vi "New Project.vi"(9 "DBSet":T1={"Server"="172.20.23.107", "DB"="HTPSDB", "PSW"="data'songyy", "User"="sa"}, 10 "UserID":string="L043460", 11 "厂区":string="清溪") -> ()   [LabVIEW 2011] (continued)
      n38 = call "Delete empty element from array.vi"("Array In"=w75) -> ("Array out"=w39:string[])  [unwired: 26 in]
      "Single init" <- w39
      n39 = call "Delete empty element from array.vi"("Array In"=w74) -> ("Array out"=w38:string[])  [unwired: 26 in]
      "TDR init" <- w38
      n40 = call "Delete empty element from array.vi"("Array In"=w73) -> ("Array out"=w37:string[])  [unwired: 26 in]
      "S-p init" <- w37
      n41 = call "Delete empty element from array.vi"("Array In"=w72) -> ("Array out"=w36:string[])  [unwired: 26 in]
      "NEXT init" <- w36
      n42 = call "Delete empty element from array.vi"("Array In"=w64) -> ("Array out"=w35:string[])  [unwired: 26 in]
      "FEXT init" <- w35
      n43 = Array Size(array=w69) -> (size(s)=w90:i32)
      n44 = Array Size(array=w39) -> (size(s)=w87:i32)
      n45 = Array Size(array=w38) -> (size(s)=w63:i32)
      n46 = Array Size(array=w37) -> (size(s)=w70:i32)
      n47 = Array Size(array=w36) -> (size(s)=w88:i32)
      n48 = Array Size(array=w35) -> (size(s)=w71:i32)
      n49 = property on="Postion for Raw data" class="Tbl (严格)"("Value"=string[][] [] ("Postion for Raw data")) -> ()  [unwired: 2 in, 2 out]
      n50 = Initialize Array(w62, w90) -> (w54:i32[])
      "Diff init" <- w54
      n51 = Initialize Array(w62, w87) -> (w53:i32[])
      "Single init" <- w53
      n52 = Initialize Array(w62, w63) -> (w52:i32[])
      "TDR init" <- w52
      n53 = Initialize Array(w62, w70) -> (w89:i32[])
      "S-p init" <- w89
      n54 = Initialize Array(w62, w88) -> (w51:i32[])
      "NEXT init" <- w51
      n55 = Initialize Array(w62, w71) -> (w50:i32[])
      "FEXT init" <- w50
      n56 = property on="Diff Test Items" class="LstBox (严格)"("Item Names"=w69, "Item Symbols"=w54) -> ()  [unwired: 2 in, 2 out]
      n57 = property on="Single Test Items" class="LstBox (严格)"("Item Names"=w39, "Item Symbols"=w53) -> ()  [unwired: 2 in, 2 out]
      n58 = property on="TDR Test Items" class="LstBox (严格)"("Item Names"=w38, "Item Symbols"=w52) -> ()  [unwired: 2 in, 2 out]
      n59 = property on="S-para Pair Name" class="LstBox (严格)"("Item Names"=w37, "Item Symbols"=w89) -> ()  [unwired: 2 in, 2 out]
      n60 = property on="NEXT Pair Name" class="LstBox (严格)"("Item Names"=w36, "Item Symbols"=w51) -> ()  [unwired: 2 in, 2 out]
      n61 = property on="FEXT Pair Name" class="LstBox (严格)"("Item Names"=w35, "Item Symbols"=w50) -> ()  [unwired: 2 in, 2 out]
      n62 = property on="访问DB(s)" class="DigNum (严格)"("Visible"=TRUE ("可见")) -> ()  [unwired: 2 in, 2 out]
      n63 = local write "fre-save"(string[] [] ("fre-save")) -> ()
      n64 = Get Date/Time In Seconds() -> (seconds since 1Jan1904=→"midVar_timeStart":timestamp)
      n65 = local write "EEPROM Write/Read ?"(w60) -> ()
      n66 = local write "Label Print?"(w60) -> ()
      n67 = local write "Report Templete Path:"(path "" ("Report Templete Path:")) -> ()
      n68 = property on="Postion for \"PN&Tester&Date\" etc Fields" class="Tbl (严格)"("Value"=string[][] [["Applicant", "0", "2", "1"], ["Part Name", "0", "3", "1"], ["Part Number", "0", "4", "1"], ["Report No", "0", "2", "12"], ["Sample No", "0", "4", "12"], ["Prepared By", "0", "63", "0"], ["Approved By", "0", "63", "6"], ["Date", "0", "63", "2"], ["Thru Result", "0", "13", "5"], ["NEXT Result", "0", "45", "4"], ["FEXT Result", "0", "45", "5"]] ("Postion for \"PN&Tester&Date\" etc Fields")) -> ()  [unwired: 2 in, 2 out]
      n69 = property on="Postion for Raw data" class="Tbl (严格)"("Number of Columns"=w59, "EditPos"=w58) -> ()  [unwired: 2 in, 2 out]
      n70 = property on="Postion for \"PN&Tester&Date\" etc Fields" class="Tbl (严格)"("Number of Columns"=w59, "EditPos"=w58) -> ()  [unwired: 2 in, 2 out]
      n71 = local write "Spec Points"(1601.0 ("Spec Points")) -> ()
      n72 = local write "Quick"(FALSE ("Quick")) -> ()
      n73 = local write "Spec Associate"(string[][] [] ("Spec Associate")) -> ()
      n74 = property on="Diff Test Items" class="LstBox (严格)"("Value"=w57) -> ()  [unwired: 2 in, 2 out]
      n75 = property on="S-para Pair Name" class="LstBox (严格)"("Value"=w57) -> ()  [unwired: 2 in, 2 out]
      n76 = property on="NEXT Pair Name" class="LstBox (严格)"("Value"=w57) -> ()  [unwired: 2 in, 2 out]
      n77 = property on="FEXT Pair Name" class="LstBox (严格)"("Value"=w57) -> ()  [unwired: 2 in, 2 out]
      n78 = property on="Single Test Items" class="LstBox (严格)"("Value"=w57) -> ()  [unwired: 2 in, 2 out]
      n79 = property on="FEXT Pair Name" class="LstBox (严格)"("Value"=w57) -> ()  [unwired: 2 in, 2 out]
      n80 = property on="Cable AWG:" class="Ring (严格)"("Value"=w57) -> ()  [unwired: 2 in, 2 out]
      n81 = property on="Customer" class="Ring (严格)"("Value"=w57) -> ()  [unwired: 2 in, 2 out]
      n82 = property on="TDR Test Items" class="LstBox (严格)"("Value"=w57) -> ()  [unwired: 2 in, 2 out]
      n83 = call <vilib>:"Application Directory.vi"() -> ("Application Directory"=w33:path)
      n84 = property on="Default" class="RadioBtnsControl (严格)"("Value"=w57) -> ()  [unwired: 2 in, 2 out]
      n85 = Build Path(base path=w33, name or relative path="template" ("名称或相对路径")) -> (appended path=w34:path)
      n86 = call "Get_initialize_Config.vi"() -> ("Local Database"=w25:bool)  [unwired: 11 in]
      n87 = local write "Report Templete Path:"(w34) -> ()
      n88 = local write "Local"(w25) -> ()
      n89 = property on="Excute" class="Bool"("DisabledEnum"=w30) -> ()  [unwired: 2 in, 2 out]
      n90 = property on="Query" class="Bool (严格)"("DisabledEnum"=w30) -> ()  [unwired: 2 in, 2 out]
      n91 = property on="Save" class="Bool (严格)"("DisabledEnum"=T5."Disabled and Grayed Out" ("禁用")) -> ()  [unwired: 2 in, 2 out]
      n92 = local write "Save"(FALSE ("Query")) -> ()
      n93 = local write "Delete"(FALSE ("Query")) -> ()
      n94 = local write "Query"(FALSE ("Query")) -> ()
      n95 = local write "Update"(FALSE ("Query")) -> ()
      n96 = property on="SNType" class="Str"("Visible"=w25) -> ()  [unwired: 2 in, 2 out]
      n97 = property on="CmdType" class="Ring (严格)"("Visible"=w25) -> ()  [unwired: 2 in, 2 out]
      n98 = property on="Update" class="Bool (严格)"("DisabledEnum"=T5."Disabled and Grayed Out" ("禁用")) -> ()  [unwired: 2 in, 2 out]
      n99 = property on="Delete" class="Bool (严格)"("DisabledEnum"=T5."Disabled and Grayed Out" ("禁用")) -> ()  [unwired: 2 in, 2 out]
      n100 = property on="Luxshare_P/N:" class="Str"("DisabledEnum"=T5."Disabled and Grayed Out" ("禁用")) -> ()  [unwired: 2 in, 2 out]
      "midVar_bool_timStop" <- FALSE ("midVar_bool_timStop")
    }
    frame #2 {
      n101 = while {
        stop <- w103 stop-if-true
        n102 = local read "midVar_timeStart"() -> (w102:timestamp)
        n103 = local read "midVar_bool_timStop"() -> (w103:bool)
        n104 = Get Date/Time In Seconds() -> (seconds since 1Jan1904=w104:timestamp)
        n105 = Subtract(x=w104, y=w102) -> (x-y=→"访问DB(s)":dbl)
      }
      n106 = call <vilib>:"System Exec.vi"("run minimized? (F)"=TRUE, "wait until completion? (T)"=TRUE, "command line"="ping DG-MESDB.luxshare.com.cn") -> ("standard output"=w95:string)  [unwired: 5 in, 3 out]
      n107 = Search and Replace String(replace all?=TRUE ("替换全部？(F)"), case sensitive?=TRUE ("忽略大小写？(F)"), input string=w95, search string="TTL" ("搜索字符串")) -> (number of replacements=w97:i32)  [unwired: 4 in, 3 out]
      n108 = Greater Than 0?(x=w97) -> (x > 0?=w92:bool)
      n109 = case shown="真" w92 {
        tunnel: "DBSet" -> [_ w112]
        frame False {
          w108 = T5."Enabled" ("禁用")
          # "连不上数据库，local禁用，默认勾选"
          n110 = property on="Query" class="Bool (严格)"("DisabledEnum"=w108) -> ()  [unwired: 2 in, 2 out]
          n111 = property on="Save" class="Bool (严格)"("DisabledEnum"=w108) -> ()  [unwired: 2 in, 2 out]
          n112 = local write "midVar_bool_timStop"(TRUE ("midVar_bool_timStop")) -> ()
          n113 = One Button Dialog(message="fail to connect DB!\nyou can use local DB only!") -> ()  [unwired: 1 in, 1 out]
          n114 = property on="Excute" class="Bool"("DisabledEnum"=w108) -> ()  [unwired: 2 in, 2 out]
          n115 = local write "Local"(TRUE ("Local")) -> ()
          n116 = property on="Local" class="Bool (严格)"("DisabledEnum"=T5."Disabled and Grayed Out" ("禁用")) -> ()  [unwired: 2 in, 2 out]
          n117 = property on="FixtureNo" class="CmbBox"("Strings And Values[]"=T6 [{"String"="No Data", "Value"="No Data"}] ("字符串与值[]")) -> ()  [unwired: 2 in, 2 out]
          n118 = property on="FixtureNo" class="CmbBox"("DisabledEnum"=T5."Disabled and Grayed Out" ("禁用")) -> ()  [unwired: 2 in, 2 out]
        }
        frame True {
          n119 = stacked-sequence {
            tunnel: w112 -> [_ w115 _]
            frame #0 {
              w114 = T5."Enabled" ("禁用")
              w113 = T5."Enabled" ("禁用")
              n120 = property on="Local" class="Bool (严格)"("DisabledEnum"=w113) -> ()  [unwired: 2 in, 2 out]
              n121 = property on="Query" class="Bool (严格)"("DisabledEnum"=w113) -> ()  [unwired: 2 in, 2 out]
              n122 = property on="Save" class="Bool (严格)"("DisabledEnum"=w114) -> ()  [unwired: 2 in, 2 out]
              n123 = property on="Excute" class="Bool"("DisabledEnum"=w114) -> ()  [unwired: 2 in, 2 out]
            }
            frame #1 {
              n124 = disable-structure shown="禁用" {
                disable-tunnel: w115 -> [w116 _]
                frame Disabled {
                  n125 = call "sql-readinfo_vproject.vi"("DBSet"=w116, "操作模式"=T7."查询数据", "查询项目"="FixtureNo", "限定条件"="") -> ("ConvertToArray"=w118:string[][], "ResultString"=w117:string)  [unwired: 13 in, 9 out]
                  n126 = call <vilib>:"Trim Whitespace.vi"("string"=w117) -> ("trimmed string"=w123:string)  [unwired: 1 in]
                  n127 = Empty String/Path?(string/path=w123) -> (empty?=w122:bool)
                  n128 = case shown="假" w122 {
                    tunnel: w118 -> [w128 _]
                    frame False {
                      n129 = Index Array(array=w128, index (col)=0 ("索引 (行)")) -> (element=w127:string[])  [unwired: 1 in]
                      n130 = for {
                        tunnel: w127 -> [w130] mode=indexing
                        tunnel: [w129] -> w126 mode=indexing
                        n131 = Bundle("字符串"=w130, "字符串"=w130) -> (w129:cluster{"字符串":string, "字符串":string})  [unwired: 1 in]
                      }
                      n132 = property on="FixtureNo" class="CmbBox"("Strings And Values[]"=w126) -> ()  [unwired: 2 in, 2 out]
                      n133 = property on="FixtureNo" class="CmbBox"("DisabledEnum"=T5."Enabled" ("禁用")) -> ()  [unwired: 2 in, 2 out]
                    }
                    frame True {
                      n134 = property on="FixtureNo" class="CmbBox"("Strings And Values[]"=T6 [{"String"="No Data", "Value"="No Data"}] ("字符串与值[]")) -> ()  [unwired: 2 in, 2 out]
                      n135 = property on="FixtureNo" class="CmbBox"("DisabledEnum"=T5."Disabled and Grayed Out" ("禁用")) -> ()  [unwired: 2 in, 2 out]
                    }
                  }
                }
                frame Enabled {
                }
              }
            }
            frame #2 {
              n136 = local write "midVar_bool_timStop"(TRUE ("midVar_bool_timStop")) -> ()
            }
          }
        }
      }
    }
    frame #3 {
      n137 = control-ref of="Label Num"() -> (w141:refnum<vi>)
      n138 = control-ref of="FixtureNo"() -> (w163:refnum<vi>)
      n139 = control-ref of="Label Num"() -> (w162:refnum<vi>)
      n140 = control-ref of="Label Content"() -> (w161:refnum<vi>)
      n141 = control-ref of="SNType"() -> (w160:refnum<vi>)
      n142 = control-ref of="Customer_P/N:"() -> (w170:refnum<vi>)
      n143 = control-ref of="Length(mm):"() -> (w169:refnum<vi>)
      n144 = control-ref of="Sample Description:"() -> (w168:refnum<vi>)
      n145 = control-ref of="Remark:"() -> (w167:refnum<vi>)
      n146 = control-ref of="Switch Matrix"() -> (w166:refnum<vi>)
      n147 = control-ref of="VNA Cal File Path:"() -> (w164:refnum<vi>)
      n148 = control-ref of="EEPROM Write/Read ?"() -> (w159:refnum<vi>)
      n149 = control-ref of="Label Print?"() -> (w158:refnum<vi>)
      n150 = Build Array(w159, w158) -> (→"bool":refnum<vi>[])
      n151 = call <vilib>:"Application Directory.vi"() -> ("Application Directory"=w137:path)
      n152 = Build Array(w164, w170, w169, w168, w167, w166, w163, w162, w161, w141, w160) -> (→"string":refnum<vi>[])
      n153 = Build Path(base path=w137, name or relative path="Database" ("名称或相对路径")) -> (appended path=w140:path)
      n154 = Build Path(base path=w140, name or relative path="FigoConfig.xml" ("名称或相对路径")) -> (appended path=w136:path)
      n155 = control-ref of="Postion for Raw data"() -> (w156:refnum<vi>)
      n156 = control-ref of="Impedance Spec:"() -> (w142:refnum<vi>)
      n157 = control-ref of="Start TimeNs"() -> (w155:refnum<vi>)
      n158 = control-ref of="StopTimeNs"() -> (w154:refnum<vi>)
      n159 = control-ref of="Filter Risetime(ps)"() -> (w153:refnum<vi>)
      n160 = control-ref of="Compensation(ohm)"() -> (w152:refnum<vi>)
      n161 = call <vilib>:"Check if File or Folder Exists.vi"("path"=w136) -> ("file or folder exists?"=w135:bool, "dup path"=w134:path)  [unwired: 8 in, 1 out]
      n162 = Build Array(w142, w156) -> (→"chart":refnum<vi>[])
      n163 = Build Array(w155, w154, w153, w152) -> (→"number":refnum<vi>[])
      n164 = case shown="真" w135 {
        tunnel: w134 -> [_ w173]
        frame False {
        }
        frame True {
          n165 = call "xmlConfigRead.vi"("path to XML document"=w173, "XPath expression"="//AWG/item/@value") -> ("OutParaArray"=w172:string[])  [unwired: 2 out]
          n166 = property on="Cable AWG:" class="Ring (严格)"("Strings []"=w172) -> ()  [unwired: 2 in, 2 out]
        }
      }
      n167 = control-ref of="Diff Test Items"() -> (w151:refnum<vi>)
      n168 = control-ref of="Single Test Items"() -> (w150:refnum<vi>)
      n169 = control-ref of="TDR Test Items"() -> (w149:refnum<vi>)
      n170 = control-ref of="S-para Pair Name"() -> (w148:refnum<vi>)
      n171 = control-ref of="NEXT Pair Name"() -> (w147:refnum<vi>)
      n172 = control-ref of="FEXT Pair Name"() -> (w146:refnum<vi>)
      n173 = Build Array(w151, w150, w149, w148, w147, w146) -> (→"list":refnum<vi>[])
      n174 = property on="访问DB(s)" class="DigNum (严格)"("Visible"=FALSE ("可见")) -> ()  [unwired: 2 in, 2 out]
    }
    frame #4 {
      n175 = while {
        stop <- w176 stop-if-true
        n176 = event shown="[17] \"Excute\": 值改变" {
          selector: _ -> [_ _ _ _ _ _ _ _ _ _ _ _ _ _ _ _ _ _ _ _ _ _ _]
          dyn-events: _ -> [_ _ _ _ _ _ _ _ _ _ _ _ _ _ _ _ _ _ _ _ _ _ _]
          timeout: 500 -> [_ _ _ _ _ _ _ _ _ _ _ _ _ _ _ _ _ _ _ _ _ _ _]
          tunnel: [_ _ _ _ _ _ _ _ _ _ _ _ _ _ _ _ _ _ _ TRUE _ _ _] -> w176
          event Timeout {
            n177 = event-data() -> ()  [unwired: 1 in, 2 out]
          }
          event "Length(mm):", "VNA Cal File Path:", "Switch Matrix", "Luxshare_P/N:": Value Change {
            n178 = event-data() -> ()  [unwired: 1 in, 5 out]
          }
          event "Local": Value Change {
            n179 = event-data() -> ()  [unwired: 1 in, 5 out]
            n180 = local read "Local"() -> (w177:bool)
            n181 = Not(x=w177) -> (.not. x?=w178:bool)
            n182 = property on="SNType" class="Str"("Visible"=w177) -> ()  [unwired: 2 in, 2 out]
            n183 = property on="CmdType" class="Ring (严格)"("Visible"=w177) -> ()  [unwired: 2 in, 2 out]
            n184 = property on="System_Mode" class="Ring (严格)"("Visible"=w178) -> ()  [unwired: 2 in, 2 out]
          }
          event "Quick": Value Change {
            n185 = event-data() -> ("NewVal"=w181:bool)  [unwired: 1 in, 4 out]
            n186 = Equal?(x=w181, y=TRUE) -> (x = y?=w179:bool)
            n187 = case shown="真" w179 {
              frame False {
                n188 = property on="Postion for Raw data" class="Tbl (严格)"("Value"=string[][] [] ("Postion for Raw data")) -> ()  [unwired: 2 in, 2 out]
              }
              frame True {
                w184 = T4 {"Row"=0, "Column"=0} ("编辑位置")
                w185 = u32 4 ("列数")
                n189 = property on="Single Test Items" class="LstBox (严格)"() -> ("Item Names"=w202:string[], "Item Symbols"=w201:i32[])  [unwired: 2 in, 2 out]
                n190 = property on="TDR Test Items" class="LstBox (严格)"() -> ("Item Names"=w200:string[], "Item Symbols"=w199:i32[])  [unwired: 2 in, 2 out]
                n191 = property on="Diff Test Items" class="LstBox (严格)"() -> ("Item Names"=w204:string[], "Item Symbols"=w203:i32[])  [unwired: 2 in, 2 out]
                n192 = call "_wmg_SelectItems2.vi"("Item Syms"=w199, "Item name"=w200) -> ("Selected tem"=w198:string[])  [unwired: 7 in, 2 out]
                n193 = call "_wmg_SelectItems2.vi"("Item Syms"=w203, "Item name"=w204) -> ("Selected tem"=w197:string[])  [unwired: 7 in, 2 out]
                n194 = call "_wmg_SelectItems2.vi"("Item Syms"=w201, "Item name"=w202) -> ("Selected tem"=w196:string[])  [unwired: 7 in, 2 out]
                n195 = Insert Into Array(array=w198, new element #1=w197, new element #2=w196) -> (w193:string[])  [unwired: 1 in]
                n196 = Array Size(array=w193) -> (size(s)=w190:i32)
                n197 = for {
                  N: w190 -> [_]
                  tunnel: [w205] -> w194 mode=indexing
                  i -> [w206]
                  n198 = Increment(x=w206) -> (x+1=w205:i32)
                }
                n199 = Initialize Array("2", w190) -> (w188:string[])
                n200 = Initialize Array("0", w190) -> (w187:string[])
                n201 = Number To Decimal String(number=w194) -> (decimal integer string=w192:string[])  [unwired: 1 in]
                n202 = Build Array(w193, w192, w188, w187) -> (w186:string[][])
                n203 = Transpose 2D Array(2D array=w186) -> (transposed array=w195:string[][])
                n204 = property on="Postion for Raw data" class="Tbl (严格)"("Value"=w195, "EditPos"=T4 {"Row"=0, "Column"=0} ("编辑位置")) -> ()  [unwired: 2 in, 2 out]
                n205 = property on="Postion for Raw data" class="Tbl (严格)"("Number of Columns"=w185, "EditPos"=w184) -> ()  [unwired: 2 in, 2 out]
                n206 = property on="Postion for \"PN&Tester&Date\" etc Fields" class="Tbl (严格)"("Number of Columns"=w185, "EditPos"=w184) -> ()  [unwired: 2 in, 2 out]
              }
            }
          }
          event "Diff Test Items": Double Click {
            n207 = event-data() -> ("Row"=w207:i32)  [unwired: 1 in, 7 out]
            n208 = stacked-sequence {
              tunnel: w207 -> [w211 _ _]
              frame #0 {
                n209 = property on="Diff Test Items" class="LstBox (严格)"() -> ("Item Symbols"=w212:i32[])  [unwired: 2 in, 2 out]
                n210 = Index Array(array=w212, index=w211) -> (element=w209:i32)
                n211 = case shown="38" w209 {
                  tunnel: [37 38 17] -> w208
                  frame 17 {
                  }
                  frame 37, Default {
                  }
                  frame 38 {
                  }
                }
                n212 = Replace Array Subset(array=w212, new element=w208, index=w211) -> (w210:i32[])
                n213 = property on="Diff Test Items" class="LstBox (严格)"("Item Symbols"=w210) -> ()  [unwired: 2 in, 2 out]
              }
              frame #1 {
                n214 = property on="Postion for Raw data" class="Tbl (严格)"("Value"=string[][] [] ("Postion for Raw data"), "EditPos"=T4 {"Row"=0, "Column"=0} ("编辑位置")) -> ()  [unwired: 2 in, 2 out]
              }
              frame #2 {
                w219 = T4 {"Row"=0, "Column"=0} ("编辑位置")
                w220 = u32 4 ("列数")
                n215 = property on="Single Test Items" class="LstBox (严格)"() -> ("Item Names"=w237:string[], "Item Symbols"=w236:i32[])  [unwired: 2 in, 2 out]
                n216 = property on="TDR Test Items" class="LstBox (严格)"() -> ("Item Names"=w235:string[], "Item Symbols"=w234:i32[])  [unwired: 2 in, 2 out]
                n217 = property on="Diff Test Items" class="LstBox (严格)"() -> ("Item Names"=w239:string[], "Item Symbols"=w238:i32[])  [unwired: 2 in, 2 out]
                n218 = property on="Postion for Raw data" class="Tbl (严格)"("Number of Columns"=w220, "EditPos"=w219) -> ()  [unwired: 2 in, 2 out]
                n219 = property on="Postion for \"PN&Tester&Date\" etc Fields" class="Tbl (严格)"("Number of Columns"=w220, "EditPos"=w219) -> ()  [unwired: 2 in, 2 out]
                n220 = call "_wmg_SelectItems2.vi"("Item Syms"=w234, "Item name"=w235) -> ("Selected tem"=w233:string[])  [unwired: 7 in, 2 out]
                n221 = call "_wmg_SelectItems2.vi"("Item Syms"=w238, "Item name"=w239) -> ("Selected tem"=w232:string[])  [unwired: 7 in, 2 out]
                n222 = call "_wmg_SelectItems2.vi"("Item Syms"=w236, "Item name"=w237) -> ("Selected tem"=w231:string[])  [unwired: 7 in, 2 out]
                n223 = Insert Into Array(array=w233, new element #1=w232, new element #2=w231) -> (w228:string[])  [unwired: 1 in]
                n224 = Array Size(array=w228) -> (size(s)=w225:i32)
                n225 = for {
                  N: w225 -> [_]
                  tunnel: [w240] -> w229 mode=indexing
                  i -> [w241]
                  n226 = Increment(x=w241) -> (x+1=w240:i32)
                }
                n227 = Initialize Array("2", w225) -> (w223:string[])
                n228 = Initialize Array("0", w225) -> (w222:string[])
                n229 = Number To Decimal String(number=w229) -> (decimal integer string=w227:string[])  [unwired: 1 in]
                n230 = Build Array(w228, w227, w223, w222) -> (w221:string[][])
                n231 = Transpose 2D Array(2D array=w221) -> (transposed array=w230:string[][])
                n232 = property on="Postion for Raw data" class="Tbl (严格)"("Value"=w230, "EditPos"=T4 {"Row"=0, "Column"=0} ("编辑位置")) -> ()  [unwired: 2 in, 2 out]
              }
            }
          }
          event "TDR Test Items": Double Click {
            n233 = event-data() -> ("Row"=w242:i32)  [unwired: 1 in, 7 out]
            n234 = stacked-sequence {
              tunnel: w242 -> [w250 _ _]
              frame #0 {
                w247 = 38 ("y")
                n235 = property on="TDR Test Items" class="LstBox (严格)"() -> ("Item Symbols"=w244:i32[])  [unwired: 2 in, 2 out]
                n236 = Index Array(array=w244, index=w250) -> (element=w249:i32)
                n237 = Equal?(x=w249, y=w247) -> (x = y?=w248:bool)
                n238 = Select(t=37, s=w248, f=w247) -> (s? t:f=w245:i32)
                n239 = Replace Array Subset(array=w244, new element=w245, index=w250) -> (w243:i32[])
                n240 = property on="TDR Test Items" class="LstBox (严格)"("Item Symbols"=w243) -> ()  [unwired: 2 in, 2 out]
              }
              frame #1 {
                n241 = property on="Postion for Raw data" class="Tbl (严格)"("Value"=string[][] [] ("Postion for Raw data"), "EditPos"=T4 {"Row"=0, "Column"=0} ("编辑位置")) -> ()  [unwired: 2 in, 2 out]
              }
              frame #2 {
                w254 = T4 {"Row"=0, "Column"=0} ("编辑位置")
                w255 = u32 4 ("列数")
                n242 = property on="Single Test Items" class="LstBox (严格)"() -> ("Item Names"=w272:string[], "Item Symbols"=w271:i32[])  [unwired: 2 in, 2 out]
                n243 = property on="TDR Test Items" class="LstBox (严格)"() -> ("Item Names"=w270:string[], "Item Symbols"=w269:i32[])  [unwired: 2 in, 2 out]
                n244 = property on="Diff Test Items" class="LstBox (严格)"() -> ("Item Names"=w274:string[], "Item Symbols"=w273:i32[])  [unwired: 2 in, 2 out]
                n245 = property on="Postion for Raw data" class="Tbl (严格)"("Number of Columns"=w255, "EditPos"=w254) -> ()  [unwired: 2 in, 2 out]
                n246 = property on="Postion for \"PN&Tester&Date\" etc Fields" class="Tbl (严格)"("Number of Columns"=w255, "EditPos"=w254) -> ()  [unwired: 2 in, 2 out]
                n247 = call "_wmg_SelectItems2.vi"("Item Syms"=w269, "Item name"=w270) -> ("Selected tem"=w268:string[])  [unwired: 7 in, 2 out]
                n248 = call "_wmg_SelectItems2.vi"("Item Syms"=w273, "Item name"=w274) -> ("Selected tem"=w267:string[])  [unwired: 7 in, 2 out]
                n249 = call "_wmg_SelectItems2.vi"("Item Syms"=w271, "Item name"=w272) -> ("Selected tem"=w266:string[])  [unwired: 7 in, 2 out]
                n250 = Insert Into Array(array=w268, new element #1=w267, new element #2=w266) -> (w263:string[])  [unwired: 1 in]
                n251 = Array Size(array=w263) -> (size(s)=w260:i32)
                n252 = for {
                  N: w260 -> [_]
                  tunnel: [w275] -> w264 mode=indexing
                  i -> [w276]
                  n253 = Increment(x=w276) -> (x+1=w275:i32)
                }
                n254 = Initialize Array("2", w260) -> (w258:string[])
                n255 = Initialize Array("0", w260) -> (w257:string[])
                n256 = Number To Decimal String(number=w264) -> (decimal integer string=w262:string[])  [unwired: 1 in]
                n257 = Build Array(w263, w262, w258, w257) -> (w256:string[][])
                n258 = Transpose 2D Array(2D array=w256) -> (transposed array=w265:string[][])
                n259 = property on="Postion for Raw data" class="Tbl (严格)"("Value"=w265, "EditPos"=T4 {"Row"=0, "Column"=0} ("编辑位置")) -> ()  [unwired: 2 in, 2 out]
              }
            }
          }
          event "S-para Pair Name": Double Click {
            w281 = 38 ("y")
            n260 = event-data() -> ("Row"=w277:i32)  [unwired: 1 in, 7 out]
            n261 = property on="S-para Pair Name" class="LstBox (严格)"() -> ("Item Symbols"=w284:i32[])  [unwired: 2 in, 2 out]
            n262 = Index Array(array=w284, index=w277) -> (element=w283:i32)
            n263 = Equal?(x=w283, y=w281) -> (x = y?=w282:bool)
            n264 = Select(t=37, s=w282, f=w281) -> (s? t:f=w279:i32)
            n265 = Replace Array Subset(array=w284, new element=w279, index=w277) -> (w278:i32[])
            n266 = property on="S-para Pair Name" class="LstBox (严格)"("Item Symbols"=w278) -> ()  [unwired: 2 in, 2 out]
          }
          event "NEXT Pair Name": Double Click {
            w289 = 38 ("y")
            n267 = event-data() -> ("Row"=w285:i32)  [unwired: 1 in, 7 out]
            n268 = property on="NEXT Pair Name" class="LstBox (严格)"() -> ("Item Symbols"=w292:i32[])  [unwired: 2 in, 2 out]
            n269 = Index Array(array=w292, index=w285) -> (element=w291:i32)
            n270 = Equal?(x=w291, y=w289) -> (x = y?=w290:bool)
            n271 = Select(t=37, s=w290, f=w289) -> (s? t:f=w287:i32)
            n272 = Replace Array Subset(array=w292, new element=w287, index=w285) -> (w286:i32[])
            n273 = property on="NEXT Pair Name" class="LstBox (严格)"("Item Symbols"=w286) -> ()  [unwired: 2 in, 2 out]
          }
          event "FEXT Pair Name": Double Click {
            w293 = 38 ("y")
            n274 = event-data() -> ("Row"=w294:i32)  [unwired: 1 in, 7 out]
            n275 = property on="FEXT Pair Name" class="LstBox (严格)"() -> ("Item Symbols"=w300:i32[])  [unwired: 2 in, 2 out]
            n276 = Index Array(array=w300, index=w294) -> (element=w299:i32)
            n277 = Equal?(x=w299, y=w293) -> (x = y?=w298:bool)
            n278 = Select(t=37, s=w298, f=w293) -> (s? t:f=w296:i32)
            n279 = Replace Array Subset(array=w300, new element=w296, index=w294) -> (w295:i32[])
            n280 = property on="FEXT Pair Name" class="LstBox (严格)"("Item Symbols"=w295) -> ()  [unwired: 2 in, 2 out]
          }
          event "Single Test Items": Double Click {
            n281 = event-data() -> ("Row"=w301:i32)  [unwired: 1 in, 7 out]
            n282 = stacked-sequence {
              tunnel: w301 -> [w303 _ _]
              frame #0 {
                w302 = 38 ("y")
                n283 = property on="Single Test Items" class="LstBox (严格)"() -> ("Item Symbols"=w309:i32[])  [unwired: 2 in, 2 out]
                n284 = Index Array(array=w309, index=w303) -> (element=w308:i32)
                n285 = Equal?(x=w308, y=w302) -> (x = y?=w307:bool)
                n286 = Select(t=37, s=w307, f=w302) -> (s? t:f=w305:i32)
                n287 = Replace Array Subset(array=w309, new element=w305, index=w303) -> (w304:i32[])
                n288 = property on="Single Test Items" class="LstBox (严格)"("Item Symbols"=w304) -> ()  [unwired: 2 in, 2 out]
              }
              frame #1 {
                n289 = property on="Postion for Raw data" class="Tbl (严格)"("Value"=string[][] [] ("Postion for Raw data"), "EditPos"=T4 {"Row"=0, "Column"=0} ("编辑位置")) -> ()  [unwired: 2 in, 2 out]
              }
              frame #2 {
                w313 = T4 {"Row"=0, "Column"=0} ("编辑位置")
                w314 = u32 4 ("列数")
                n290 = property on="Single Test Items" class="LstBox (严格)"() -> ("Item Names"=w331:string[], "Item Symbols"=w330:i32[])  [unwired: 2 in, 2 out]
                n291 = property on="TDR Test Items" class="LstBox (严格)"() -> ("Item Names"=w329:string[], "Item Symbols"=w328:i32[])  [unwired: 2 in, 2 out]
                n292 = property on="Diff Test Items" class="LstBox (严格)"() -> ("Item Names"=w333:string[], "Item Symbols"=w332:i32[])  [unwired: 2 in, 2 out]
                n293 = property on="Postion for Raw data" class="Tbl (严格)"("Number of Columns"=w314, "EditPos"=w313) -> ()  [unwired: 2 in, 2 out]
                n294 = property on="Postion for \"PN&Tester&Date\" etc Fields" class="Tbl (严格)"("Number of Columns"=w314, "EditPos"=w313) -> ()  [unwired: 2 in, 2 out]
                n295 = call "_wmg_SelectItems2.vi"("Item Syms"=w328, "Item name"=w329) -> ("Selected tem"=w327:string[])  [unwired: 7 in, 2 out]
                n296 = call "_wmg_SelectItems2.vi"("Item Syms"=w332, "Item name"=w333) -> ("Selected tem"=w326:string[])  [unwired: 7 in, 2 out]
                n297 = call "_wmg_SelectItems2.vi"("Item Syms"=w330, "Item name"=w331) -> ("Selected tem"=w325:string[])  [unwired: 7 in, 2 out]
                n298 = Insert Into Array(array=w327, new element #1=w326, new element #2=w325) -> (w322:string[])  [unwired: 1 in]
                n299 = Array Size(array=w322) -> (size(s)=w319:i32)
                n300 = for {
                  N: w319 -> [_]
                  tunnel: [w334] -> w323 mode=indexing
                  i -> [w335]
                  n301 = Increment(x=w335) -> (x+1=w334:i32)
                }
                n302 = Initialize Array("2", w319) -> (w317:string[])
                n303 = Initialize Array("0", w319) -> (w316:string[])
                n304 = Number To Decimal String(number=w323) -> (decimal integer string=w321:string[])  [unwired: 1 in]
                n305 = Build Array(w322, w321, w317, w316) -> (w315:string[][])
                n306 = Transpose 2D Array(2D array=w315) -> (transposed array=w324:string[][])
                n307 = property on="Postion for Raw data" class="Tbl (严格)"("Value"=w324, "EditPos"=T4 {"Row"=0, "Column"=0} ("编辑位置")) -> ()  [unwired: 2 in, 2 out]
              }
            }
          }
          event "Import Spec": Value Change {
            n308 = event-data() -> ()  [unwired: 1 in, 5 out]
            n309 = case shown="真" "Import Spec" {
              frame False {
              }
              frame True {
                n310 = call <vilib>:"Application Directory.vi"() -> ("Application Directory"=w339:path)
                n311 = Build Path(base path=w339, name or relative path="Spec" ("名称或相对路径")) -> (appended path=w337:path)
                n312 = call "文件对话框"("start path"=w337) -> ("selected path"=w341:path, "error out"=w340:errorcluster)  [unwired: 11 in, 2 out]
                n313 = case shown="无错误" w340 {
                  tunnel: w341 -> [w342 _]
                  frame No Error {
                    n314 = stacked-sequence {
                      tunnel: w342 -> [_ w345]
                      frame #0 {
                      }
                      frame #1 {
                        n315 = Path To String(path=w345) -> (string=w347:string)
                        n316 = call "readLossSpecFromExcel.vi"("Spec Points"="Spec Points", "Spec Path"=w345) -> ("lossSpec"=w343:string[][])  [unwired: 8 in, 1 out]
                        n317 = Array To Spreadsheet String(delimiter (Tab)="#" ("分隔符(Tab)"), array=w343, 3:"%s" ("格式字符串")) -> (spreadsheet string=→"Spec String":string)
                        n318 = local write "Spec File Path"(w347) -> ()
                        n319 = call "offsetOverSizeJudge.vi"("lossSpec"=w343) -> ("inSpec?"=w344:bool)  [unwired: 10 in]
                        n320 = case shown="真" w344 {
                          tunnel: w343 -> [_ w351]
                          frame False {
                          }
                          frame True {
                            n321 = stacked-sequence {
                              tunnel: w351 -> [_ w353]
                              frame #0 {
                                n322 = local write "Spec Associate"(string[][] [] ("Spec Associate")) -> ()
                              }
                              frame #1 {
                                n323 = local write "Spec Associate"(w353) -> ()
                              }
                            }
                          }
                        }
                      }
                    }
                  }
                  frame Error {
                  }
                }
              }
            }
          }
          event "From File": Value Change {
            n324 = event-data() -> ()  [unwired: 1 in, 5 out]
            n325 = case shown="假" "From File" {
              tunnel: [2 0] -> w354
              frame False {
              }
              frame True {
              }
            }
            n326 = property on="Import_FixS4P" class="Bool"("DisabledEnum"=w354) -> ()  [unwired: 2 in, 2 out]
          }
          event "FixtureType": Value Change {
            n327 = event-data() -> ()  [unwired: 1 in, 5 out]
            n328 = local read "DBSet"() -> (w358:T1)
            n329 = local read "FixtureNo"() -> (w360:string)
            n330 = Search and Replace String(input string=" where FixtureNo='@' " ("限定条件"), search string="@" ("搜索字符串"), replace string=w360) -> (result string=w359:string)  [unwired: 5 in, 3 out]
            n331 = call "sql-readinfo_vfixture.vi"("DBSet"=w358, "操作模式"=T7."查询数据", "查询项目"=" S4P10G,S4P20G,S4P27G,S4P40G ", "限定条件"=w359) -> ("ConvertToArray"=w367:string[][], "ResultString"=w366:string)  [unwired: 13 in, 9 out]
            n332 = call <vilib>:"Trim Whitespace.vi"("string"=w366) -> ("trimmed string"=w365:string)  [unwired: 1 in]
            n333 = Empty String/Path?(string/path=w365) -> (empty?=w364:bool)
            n334 = case shown="假" w364 {
              tunnel: w367 -> [w373 _]
              frame False {
                n335 = Index Array(array=w373, index (col)=0 ("索引 (行)")) -> (element=w372:string[])  [unwired: 1 in]
                n336 = for {
                  tunnel: w372 -> [w375] mode=indexing
                  tunnel: [w374] -> w371 mode=indexing
                  n337 = Bundle("字符串"=w375, "字符串"=w375) -> (w374:cluster{"字符串":string, "字符串":string})  [unwired: 1 in]
                }
                n338 = property on="FixtureNo" class="CmbBox"("Strings And Values[]"=w371) -> ()  [unwired: 2 in, 2 out]
                n339 = property on="FixtureNo" class="CmbBox"("DisabledEnum"=T5."Enabled" ("禁用")) -> ()  [unwired: 2 in, 2 out]
              }
              frame True {
                n340 = property on="FixtureNo" class="CmbBox"("Strings And Values[]"=T6 [{"String"="No Data", "Value"="No Data"}] ("字符串与值[]")) -> ()  [unwired: 2 in, 2 out]
                n341 = property on="FixtureNo" class="CmbBox"("DisabledEnum"=T5."Disabled and Grayed Out" ("禁用")) -> ()  [unwired: 2 in, 2 out]
              }
            }
          }
          event "Import_FixS4P": Value Change {
            n342 = event-data() -> ()  [unwired: 1 in, 5 out]
            n343 = case shown="真" "Import_FixS4P" {
              frame False {
              }
              frame True {
                n344 = call "文件对话框3"("pattern (all files)"="*.s4p" ("DNL"), "pattern label"="SnP文件") -> ("selected path"=w380:path, "exists"=w381:bool)  [unwired: 10 in, 2 out]
                n345 = case shown="真" w381 {
                  tunnel: w380 -> [_ w385]
                  tunnel: "Port Type" -> [_ w384]
                  frame False {
                  }
                  frame True {
                    n346 = stacked-sequence {
                      tunnel: w385 -> [_ w396 w409 _]
                      tunnel: w384 -> [_ w391 w407 _]
                      frame #0 {
                        n347 = property on="Import_FixS4P" class="Bool"("DisabledEnum"=2) -> ()  [unwired: 2 in, 2 out]
                      }
                      frame #1 {
                        n348 = call "S4P to Sparameter.vi"("S4P File Path"=w396, "Port Type"=w391) -> ("Frequency(Hz)"=w393:dbl[], "Diff S-parameters Data"=w395:dbl[][])  [unwired: 14 in, 2 out]
                        n349 = Index Array(array=w395, index (row)=0 ("索引 (行)")) -> (element=w389:dbl[])  [unwired: 1 in]
                        "2X Thru  IL Data" <- w389
                        n350 = Bundle("Frequency(Hz)"=w393, "Diff S-parameters Data"=w389) -> (w392:T3)  [unwired: 1 in]
                        n351 = local write "Insertion Loss"(w392) -> ()
                        n352 = Array To Spreadsheet String(array=w389, 3:"%s" ("格式字符串")) -> (spreadsheet string=w388:string)  [unwired: 1 in]
                        n353 = call <vilib>:"Trim Whitespace.vi"("string"=w388) -> ("trimmed string"=→"2X Thru String":string)  [unwired: 1 in]
                      }
                      frame #2 {
                        w412 = i16 2 items=["StepReal", "ImpulseReal", "StepVolts", "ImpulseVolts", "StepLog", "ImpulseLog", "StepImpedance"] ("dataFormat")
                        n354 = Path To String(path=w409) -> (string=w408:string)
                        n355 = call "Export_TimeDomain_Data.vi"("szFileName"=w408, "dataFormat"=w412, "stopTimeNs"=1.6, "ParamList"="TDD21", "Port Type"=w407, "startTimeNs"=0.0) -> ("Data Out"=w406:dbl[][], "Time Array"=w399:dbl[])  [unwired: 20 in]
                        n356 = Index Array(array=w406, index (row)=0 ("索引 (行)")) -> (element=w402:dbl[])  [unwired: 1 in]
                        "2X Delay Data" <- w402
                        n357 = Threshold 1D Array(2:0.2 ("过阈值的y"), 3:w402) -> (0:w400:dbl)  [unwired: 1 in]
                        n358 = To Long Integer(number=w400) -> (32bit integer=w398:i32)
                        n359 = Bundle("Time Array"=w399, "Data Out"=w402) -> (w404:cluster{"Time Array":dbl[], "Data Out":dbl[]})  [unwired: 1 in]
                        n360 = Index Array(array=w399, index=w398) -> (element=→"Delay(ns)":dbl)
                        n361 = local write "Delay"(w404) -> ()
                      }
                      frame #3 {
                        n362 = property on="Import_FixS4P" class="Bool"("DisabledEnum"=0) -> ()  [unwired: 2 in, 2 out]
                      }
                    }
                  }
                }
              }
            }
          }
          event "Import Matrix?": Value Change {
            n363 = event-data() -> ()  [unwired: 1 in, 5 out]
            n364 = case shown="真" "Import Matrix?" {
              frame False {
              }
              frame True {
                n365 = call <vilib>:"Application Directory.vi"() -> ("Application Directory"=w417:path)
                n366 = Build Path(base path=w417, name or relative path="Switch Matrix" ("名称或相对路径")) -> (appended path=w415:path)
                n367 = call "文件对话框2"("start path"=w415) -> ("selected path"=w418:path, "error out"=w419:errorcluster)  [unwired: 11 in, 2 out]
                n368 = case shown="无错误" w419 {
                  tunnel: w418 -> [w421 _]
                  frame No Error {
                    n369 = Path To String(path=w421) -> (string=w420:string)
                    n370 = call-poly <vilib>:"Read From Spreadsheet File.vi"("format (%s)"="%s" ("format (%.3f)"), "file path (dialog if empty)"=w421) -> ("all rows"=w425:string[][])  [unwired: 5 in, 4 out]
                    n371 = Array To Spreadsheet String(delimiter (Tab)="#" ("分隔符(Tab)"), array=w425, 3:"%s" ("格式字符串")) -> (spreadsheet string=w422:string)
                    n372 = local write "Switch File Path"(w420) -> ()
                    n373 = local write "Switch Matrix"(w422) -> ()
                  }
                  frame Error {
                  }
                }
              }
            }
          }
          event "Impedance Spec:": Value Change {
            n374 = event-data() -> ()  [unwired: 1 in, 5 out]
            n375 = local read "Impedance Spec:"() -> (w427:string[][])
            n376 = call "impedance spec.vi"("Impedance Spec:"=w427) -> ("Impedance spec string"=→"Impedance spec string":string)  [unwired: 10 in]
          }
          event "Query", "Update", "Delete", "Save": Value Change {
            n377 = event-data() -> ("CtlRef"=w430:refnum<vi>)  [unwired: 1 in, 4 out]
            n378 = property class="Bool (严格)"(reference=w430) -> ("Label.Text"=w429:string)  [unwired: 1 in, 2 out]
            n379 = case shown="\"Save\"" w429 {
              frame "", Default {
                n380 = local write "Delete"(FALSE ("Delete")) -> ()
                n381 = local write "Save"(FALSE ("Save")) -> ()
                n382 = local write "Query"(FALSE ("Query")) -> ()
                n383 = local write "Update"(FALSE ("Update")) -> ()
              }
              frame "Query" {
                n384 = local write "Delete"(FALSE ("Delete")) -> ()
                n385 = local write "Save"(FALSE ("Save")) -> ()
                n386 = local write "Query"(TRUE ("Query")) -> ()
                n387 = local write "Update"(FALSE ("Update")) -> ()
                n388 = property on="Luxshare_P/N:" class="Str"("DisabledEnum"=T5."Enabled" ("禁用")) -> ()  [unwired: 2 in, 2 out]
              }
              frame "Update" {
                n389 = local write "Delete"(FALSE ("Delete")) -> ()
                n390 = local write "Save"(FALSE ("Save")) -> ()
                n391 = local write "Query"(FALSE ("Query")) -> ()
                n392 = local write "Update"(TRUE ("Update")) -> ()
                n393 = property on="Luxshare_P/N:" class="Str"("DisabledEnum"=T5."Disabled and Grayed Out" ("禁用")) -> ()  [unwired: 2 in, 2 out]
              }
              frame "Delete" {
                n394 = local write "Delete"(TRUE ("Delete")) -> ()
                n395 = local write "Save"(FALSE ("Save")) -> ()
                n396 = local write "Query"(FALSE ("Query")) -> ()
                n397 = local write "Update"(FALSE ("Update")) -> ()
                n398 = property on="Luxshare_P/N:" class="Str"("DisabledEnum"=T5."Disabled and Grayed Out" ("禁用")) -> ()  [unwired: 2 in, 2 out]
              }
              frame "Save" {
                n399 = local write "Delete"(FALSE ("Delete")) -> ()
                n400 = local write "Save"(TRUE ("Save")) -> ()
                n401 = local write "Query"(FALSE ("Query")) -> ()
                n402 = local write "Update"(FALSE ("Update")) -> ()
                n403 = property on="Luxshare_P/N:" class="Str"("DisabledEnum"=T5."Enabled" ("禁用")) -> ()  [unwired: 2 in, 2 out]
              }
            }
          }
          event "Excute": Value Change {
            n404 = event-data() -> ()  [unwired: 1 in, 5 out]
            n405 = local read "Update"() -> (w460:bool)
            n406 = local read "Delete"() -> (w458:bool)
            n407 = local read "Query"() -> (w459:bool)
            n408 = local read "Save"() -> (w457:bool)
            n409 = local read "DBSet"() -> (w455:T1)
            n410 = call "_wmg_4booltonum.vi"("input4"=w457, "input3"=w458, "input2"=w460, "input1"=w459) -> ("output"=w456:i16)
            n411 = case shown="1" w456 {
              tunnel: w455 -> [_ w461 w935 w1225 w1269]
              frame 0, Default {
              }
              frame 1000 {
                n412 = stacked-sequence {
                  tunnel: w461 -> [w462 _ _ _]
                  frame #0 {
                    n413 = local read "Local"() -> (w463:bool)
                    n414 = case shown="真" w463 {
                      tunnel: w462 -> [_ w537]
                      frame True {
                        n415 = stacked-sequence {
                          frame #0 {
                            # "从本地查询，文件一次读取，数据存放在 localQueryResult 中"
                            n416 = local read "Luxshare_P/N:"() -> (w474:string)
                            n417 = Concatenate Strings("Database\\" ("字符串"), w474, ".hpj") -> (w471:string)
                            n418 = call <vilib>:"Application Directory.vi"() -> ("Application Directory"=w472:path)
                            n419 = Build Path(base path=w472, name or relative path=w471) -> (appended path=w470:path)
                            n420 = Read from Binary File(5:string[] [], 9:T8."big-endian, network order" ("字节顺序(0:big-endian, network order)"), 11:w470) -> (0:w465:errorcluster, 2:→"localQueryResult":string[])  [unwired: 3 in, 2 out]
                            n421 = Unbundle(w465) -> ("status"=w464:bool)  [unwired: 2 out]
                            "fileexist" <- w464
                            n422 = case shown="真" w464 {
                              frame False {
                              }
                              frame True {
                                n423 = One Button Dialog(message="请检查文件是否存在") -> ()  [unwired: 1 in, 1 out]
                              }
                            }
                          }
                          frame #1 {
                            # "解析 localQueryResult"
                            n424 = local read "localQueryResult"() -> (w496:string[])
                            n425 = Index Array(array=w496, index #1=0 ("索引"), index #6=5 ("索引"), index #11=10 ("索引")) -> (element #2=w492:string, element #3=w491:string, element #4=w490:string, element #5=w489:string, element #6=w488:string, element #7=w487:string, element #8=w486:string, element #9=w485:string, element #10=w476:string, element #11=w477:string, element #12=w481:string, element #13=w480:string)  [unwired: 10 in, 1 out]
                            n426 = Decimal String To Number(string=w476) -> (number=w482:i32)  [unwired: 2 in, 1 out]
                            n427 = local write "FixtureNo"(w480) -> ()
                            n428 = local write "SNType"(w481) -> ()
                            n429 = Number To Boolean Array(number=w482) -> (Boolean array=w484:bool[])
                            n430 = Index Array(array=w484) -> (element=w483:bool)  [unwired: 1 in]
                            n431 = property on="CmdType" class="Ring (严格)"() -> ("StringsAndValues[]"=w478:T10)  [unwired: 2 in, 2 out]
                            n432 = local write "Project Information"(w490) -> ()
                            n433 = local write "Customer_P/N:"(w492) -> ()
                            n434 = local write "Sample Description:"(w489) -> ()
                            n435 = local write "Customer"(w491) -> ()
                            n436 = local write "Switch Matrix"(w485) -> ()
                            n437 = local write "Length(mm):"(w487) -> ()
                            n438 = local write "AWG"(w488) -> ()
                            n439 = local write "Spec_midVar"(w486) -> ()
                            n440 = local write "EEPROM Write/Read ?"(w483) -> ()
                            n441 = call "_wmg_downlistValue.vi"(1:"Customer"=w477, 2:"Customer"=w478) -> ("Customer"=w479:u16)
                            n442 = local write "CmdType"(w479) -> ()
                          }
                          frame #2 {
                            n443 = local read "localQueryResult"() -> (w519:string[])
                            n444 = Index Array(array=w519, index #1=13 ("索引"), index #4=16 ("索引")) -> (element #1=w513:string, element #2=w512:string, element #3=w511:string, element #4=w510:string, element #5=w506:string, element #6=w501:string, element #7=w500:string, element #8=w499:string, element #9=w498:string)  [unwired: 7 in]
                            n445 = Decimal String To Number(string=w498) -> (number=w497:i32)  [unwired: 2 in, 1 out]
                            n446 = local write "Spec File Path"(w499) -> ()
                            n447 = local write "Switch File Path"(w500) -> ()
                            n448 = Decimal String To Number(string=w513) -> (number=w514:i32)  [unwired: 2 in, 1 out]
                            n449 = local write "Label Content"(w511) -> ()
                            n450 = Decimal String To Number(string=w506) -> (number=w509:i32)  [unwired: 2 in, 1 out]
                            n451 = local write "Remark:"(w510) -> ()
                            n452 = local write "Label Num"(w512) -> ()
                            n453 = Number To Boolean Array(number=w514) -> (Boolean array=w516:bool[])
                            n454 = Number To Boolean Array(number=w509) -> (Boolean array=w508:bool[])
                            n455 = Index Array(array=w516) -> (element=w515:bool)  [unwired: 1 in]
                            n456 = Spreadsheet String To Array(delimiter (Tab)="," ("分隔符(Tab)"), format string="" ("格式字符串"), spreadsheet string=w501, array type (2D Dbl)=string[] []) -> (array=w504:string[])
                            n457 = Index Array(array=w508) -> (element=w507:bool)  [unwired: 1 in]
                            n458 = local write "fre-save"(w504) -> ()
                            n459 = local write "Label Print?"(w515) -> ()
                            n460 = local write "AutoSN"(w507) -> ()
                            n461 = local write "Spec Points"(w497) -> ()
                          }
                          frame #3 {
                            n462 = property on="Cable AWG:" class="Ring (严格)"() -> ("StringsAndValues[]"=w532:T10)  [unwired: 2 in, 2 out]
                            n463 = property on="Customer" class="Ring (严格)"() -> ("StringsAndValues[]"=w534:T10)  [unwired: 2 in, 2 out]
                            n464 = local read "Spec_midVar"() -> (w521:string)
                            n465 = local read "Customer"() -> (w533:string)
                            n466 = local read "AWG"() -> (w531:string)
                            n467 = Search and Replace String(replace all?=TRUE ("替换全部？(F)"), input string=w521, search string="#" ("搜索字符串"), replace string="\t") -> (result string=w527:string)  [unwired: 4 in, 3 out]
                            n468 = call "_wmg_downlistValue.vi"(1:"Customer"=w531, 2:"Customer"=w532) -> ("Customer"=w535:u16)
                            n469 = call "_wmg_downlistValue.vi"(1:"Customer"=w533, 2:"Customer"=w534) -> ("Customer"=w536:u16)
                            n470 = local write "Cable AWG:"(w535) -> ()
                            n471 = local write "Customer"(w536) -> ()
                            n472 = Spreadsheet String To Array(format string="%s" ("格式字符串"), spreadsheet string=w527, array type (2D Dbl)=string[][] []) -> (array=w520:string[][])  [unwired: 1 in]
                            n473 = Array To Spreadsheet String(delimiter (Tab)="#" ("分隔符(Tab)"), array=w520, 3:"%s" ("格式字符串")) -> (spreadsheet string=w522:string)
                            n474 = local write "Spec String"(w522) -> ()
                            n475 = local write "Spec Associate"(w520) -> ()
                          }
                        }
                      }
                      frame False {
                        n476 = stacked-sequence {
                          seq-local: [w557 _ _ _ _] -> [_ w583 _ _ _]
                          tunnel: w537 -> [w538 _ w584 w643 _]
                          frame #0 {
                            # "1 2 3 4 5 6 \n10 11"
                            n477 = local read "Luxshare_P/N:"() -> (w570:string)
                            n478 = property on="System_Mode" class="Ring (严格)"() -> ("RingText.Text"=w543:string)  [unwired: 2 in, 2 out]
                            n479 = local read "厂区"() -> (w539:string)
                            n480 = Array To Spreadsheet String(delimiter (Tab)="," ("分隔符(Tab)"), array=string[] ["LuxsharePN", "CustomerPN", "Customer", "SampleDes", "AWG", "Length", "EEPROMTF", "FixtureNo", "LabelTF", "LabelNum", "Remark", "AutoSN", "FrePoints", "Switch_File_Path", "Spec_File_Path", "Spec_Points", "HardWare_Mode"], 3:"" ("格式字符串")) -> (spreadsheet string=w552:string)
                            n481 = call "_wmg_PNtoPNwhereConnect.vi"("Input"=w570) -> ("Output"=w541:string)
                            n482 = call "_wmg_HardModetoHardModewhereConnect.vi"("Input"=w543, "Factory"=w539) -> ("Output"=w542:string)
                            n483 = Concatenate Strings(w541, w542) -> (w540:string)
                            n484 = call "sql-readinfo_vproject.vi"("DBSet"=w538, "操作模式"=T7."查询数据", "查询项目"=w552, "限定条件"=w540) -> ("ConvertToArray"=w569:string[][], "ResultString"=→"result_query":string)  [unwired: 13 in, 9 out]
                            n485 = Index Array(array=w569, index (row)=0 ("索引 (行)")) -> (element=w557:string[])  [unwired: 1 in]
                            n486 = Index Array(array=w557, index #1=1 ("索引"), index #6=6 ("索引")) -> (element #1=w566:string, element #2=→"Customer":string, element #3=w562:string, element #4=→"AWG":string, element #5=w561:string, element #6=w558:string, element #7=w550:string, element #8=w546:string, element #9=w545:string, element #10=w544:string)  [unwired: 8 in]
                            n487 = Decimal String To Number(string=w558) -> (number=w556:i32)  [unwired: 2 in, 1 out]
                            n488 = Decimal String To Number(string=w546) -> (number=w547:i32)  [unwired: 2 in, 1 out]
                            n489 = local write "FixtureNo"(w550) -> ()
                            n490 = local write "Remark:"(w544) -> ()
                            n491 = local write "Label Num"(w545) -> ()
                            n492 = Number To Boolean Array(number=w556) -> (Boolean array=w565:bool[])
                            n493 = Number To Boolean Array(number=w547) -> (Boolean array=w549:bool[])
                            n494 = Index Array(array=w565) -> (element=w564:bool)  [unwired: 1 in]
                            n495 = Index Array(array=w549) -> (element=w548:bool)  [unwired: 1 in]
                            n496 = local write "Customer_P/N:"(w566) -> ()
                            n497 = local write "Sample Description:"(w562) -> ()
                            n498 = local write "Length(mm):"(w561) -> ()
                            n499 = local write "EEPROM Write/Read ?"(w564) -> ()
                            n500 = local write "Label Print?"(w548) -> ()
                          }
                          frame #1 {
                            # "数据库中的cmdType不再使用，\n数据库中的SNType不再使用，代之以标签数据库中的snFormat"
                            n501 = Index Array(array=w583, index #1=11 ("索引"), index #2=12 ("索引")) -> (element #1=w579:string, element #2=w575:string)
                            n502 = Decimal String To Number(string=w579) -> (number=w580:i32)  [unwired: 2 in, 1 out]
                            n503 = Number To Boolean Array(number=w580) -> (Boolean array=w581:bool[])
                            n504 = Spreadsheet String To Array(delimiter (Tab)="," ("分隔符(Tab)"), format string="" ("格式字符串"), spreadsheet string=w575, array type (2D Dbl)=string[] []) -> (array=w574:string[])
